vi "Get Object.vi"(6 "Version ID":string, 7 "Request Parameters":T3, 8 "error in (no error)":errorcluster, 10 "Object Path":string, 11 "Bucket in":refnum<class "Bucket.lvclass">) -> (0 "error out":errorcluster, 1 "Object Info":T2, 2 "Data":string, 3 "Bucket out":refnum<class "Bucket.lvclass">, 5 "User-Defined Metadata":T1[](array[typedef]))   [LabVIEW 2015, in "NI_AWS_S3.lvlib" / "Bucket.lvclass"]
doc: "This implementation of the GET operation retrieves objects from Amazon S3. To use GET, you must have READ access to the object. If you grant READ access to the anonymous user, you can return the object without using an authorization header.\n\nAn Amazon S3 bucket has no directory hierarchy such as you would find in a typical computer file system. You can, however, create a logical hierarchy by using object key names that imply a folder structure. For example, instead of naming an object sample.jpg, you can name it photos/2006/February/sample.jpg.\n\nTo get an object from such a logical hierarchy, specify the full key name for the object in the GET operation. For a virtual hosted-style request example, if you have the object photos/2006/February/sample.jpg, specify the resource as /photos/2006/February/sample.jpg. For a path-style request example, if you have the object photos/2006/February/sample.jpg in the bucket named examplebucket, specify the resource as /examplebucket/photos/2006/February/sample.jpg."
uses:
  Bucket.lvclass
  GET Object Request Parameters.ctl
  Core/Request Range.ctl
  GET Object Result Parameters.ctl
  Core/HTTP Request/Name Value Pair.ctl
  Core/HTTP Request/Request Options.ctl
  Core/HTTP Request/Region handling.ctl
  Core/HTTP Request/URL formatting.ctl
  Bucket.lvclass/Bucket.ctl
  Read Name.vi
  Core/HTTP Request/HTTP Request.lvclass
  Object/Object.lvlib
  NI_AWS_S3.lvlib
  Core/NI_AWS_Core.lvlib
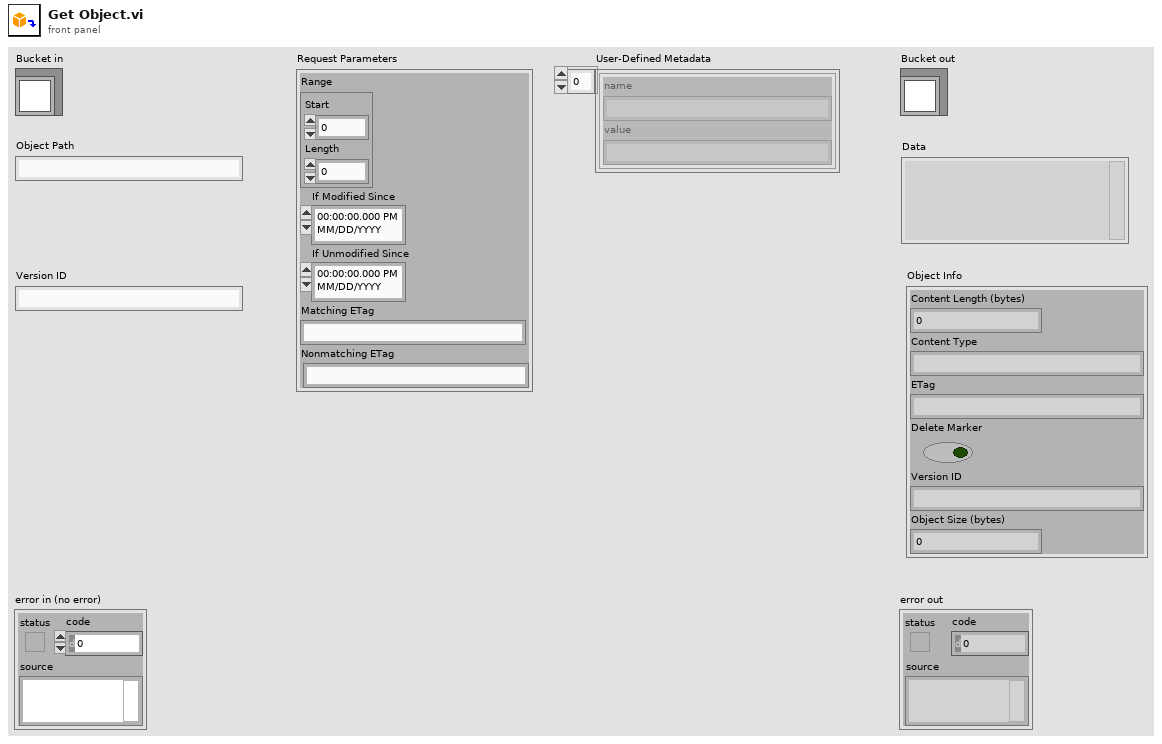
[diagram p1: front panel]
types:
  T1 = typedef "NI_AWS_Core.lvlib/HTTP Request.lvclass/Name Value Pair.ctl" = cluster{"name":string, "value":string}
  T2 = typedef "NI_AWS_S3.lvlib/GET Object Result Parameters.ctl" = cluster{"Content Length (bytes)":u64, "Content Type":string, "ETag":string, "Delete Marker":bool, "Version ID":string, "Object Size (bytes)":u64}
  T3 = typedef "NI_AWS_S3.lvlib/GET Object Request Parameters.ctl" = cluster{"Range":T4, "If Modified Since":timestamp, "If Unmodified Since":timestamp, "Matching ETag":string, "Nonmatching ETag":string}
  T4 = typedef "NI_AWS_Core.lvlib/Request Range.ctl" = cluster{"Start":i64, "Length":i64}
  T5 = typedef "NI_AWS_Core.lvlib/HTTP Request.lvclass/Region handling.ctl" = enum16{"use region everywhere", "use region (authentication only)", "use region (URL only)", "ignore region everwhere"}
  T6 = typedef "NI_AWS_Core.lvlib/HTTP Request.lvclass/Request Options.ctl" = cluster{"request headers":T1[], "request parameters":T1[], "request body":string, "region handling":T5, "URL formatting":T7}
  T7 = typedef "NI_AWS_Core.lvlib/HTTP Request.lvclass/URL formatting.ctl" = enum16{"region-", "region."}
  T8 = typedef "NI_AWS_Core.lvlib/HTTP Request.lvclass/Response.ctl" = cluster{"Headers":string, "Body":string}
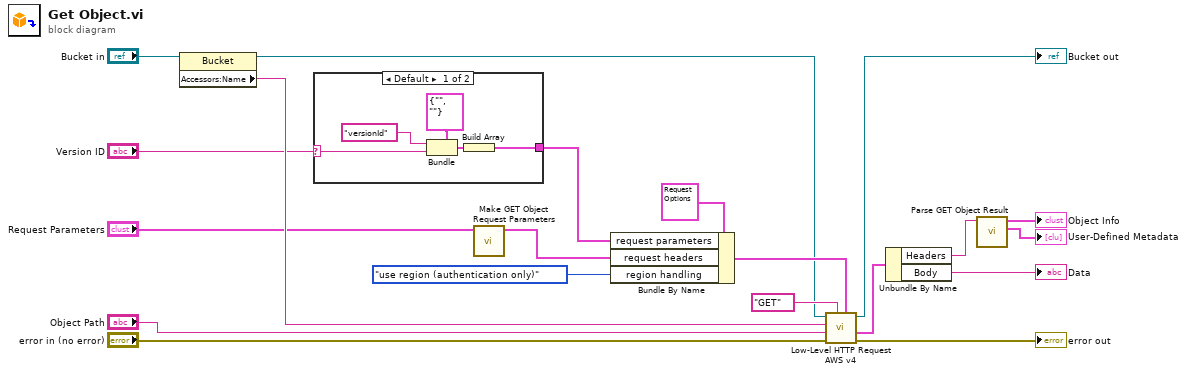
[diagram p0: block diagram]
diagram:
  n1 = property class="Bucket"(reference="Bucket in") -> (reference out=w3:refnum<class "Bucket.lvclass">, "Accessors:Name"=w19:string)  [unwired: 1 in, 1 out]
  n2 = case shown="Default" "Version ID" {
    selector: "Version ID" -> [w22 _]
    tunnel: [w23 _] -> w13
    frame Default {
      n3 = Bundle(cluster=T1 {"name"="", "value"=""} ("Name Value Pair"), "name"="versionId", "value"=w22) -> (w24:T1)
      n4 = Build Array(w24) -> (w23:T1[])
    }
    frame "" {
    }
  }
  n5 = call "Make GET Object Request Parameters.vi"("GET Object Request Parameters"="Request Parameters") -> ("HTTP Headers"=w11:T1[])  [unwired: 10 in]
  n6 = Bundle By Name(cluster=T6 {"request headers"=[], "request parameters"=[], "request body"="", "region handling"=enum."use region everywhere", "URL formatting"=enum."region."} ("Request Options"), "request parameters"=w13, "request headers"=w11, "region handling"=Region_handling."use region (authentication only)") -> (w5:T6)
  n7 = call "Low-Level HTTP Request AWS v4.vi"("Request Options"=w5, "HTTP-Verb"="GET", "error in (no error)"="error in (no error)", "URL Suffix"="Object Path", "URL Prefix"=w19, "AWS Core in"=w3) -> ("error out"=→"error out":errorcluster, "Response"=w7:T8, "AWS Core out"=→"Bucket out":refnum<class "Bucket.lvclass">)  [unwired: 2 in, 1 out]
  n8 = Unbundle By Name(w7) -> ("Headers"=w9:string, "Body"=→"Data":string)
  n9 = call "Parse GET Object Result.vi"("Response header"=w9) -> ("User-Defined Metadata"=→"User-Defined Metadata":T1[], "Get Object Result"=→"Object Info":T2)  [unwired: 9 in]
